vi "Save Image.vi"(8 "error in (no error)":errorcluster, 11 "Save Image in":refnum<class "Save Image.lvclass">) -> (0 "error out":errorcluster, 3 "Save Image out":refnum<class "Save Image.lvclass">)   [LabVIEW 2018, in "Save Image.lvclass"]
doc: "Save image using the Python Toolkit"
uses:
  Save Image.lvclass
  Save Image.lvclass/Save Image.ctl
  Log File/Log File.lvclass/Log File.ctl
  Channel/Channel.lvclass
  Log File/Log File.lvclass
  Python Toolkit/Python Toolkit.lvclass
  Sim_CCD/Sim_CCD.lvclass
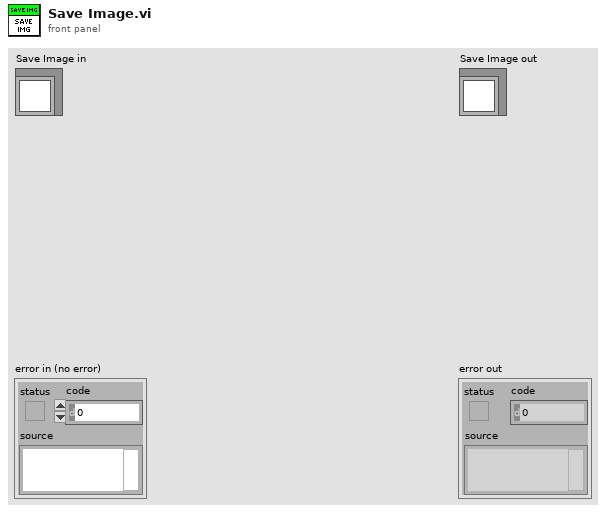
[diagram p1: front panel]
types:
  T1 = cluster{"CCD":string, "GUI":string, "ICS":string, "TCS":string, "FOCUSER":string, "WSTATION":string, "GENERAL KW":string}
  T2 = cluster{"Image path":path, "Channel":u8, "ACS mode":u16, "Log file path":path, "log level":u16}
  T3 = cluster{"CYCLES_DONE":u16, "LAST_IMAGE_NAME":string, "USED_DISK_SPACE":u16, "IMAGE_INDEX":u32, "acquisition error":bool}
  T4 = cluster{"State Machine.lvclass":refnum<class "State Machine.lvclass">, "RxTx.lvclass":refnum<class "RxTx.lvclass">, "Save_Header_RxTx.lvclass":refnum<class "RxTx.lvclass">, "Status SM.lvclass":refnum<class "State Machine.lvclass">, "Status RxTx.lvclass":refnum<class "RxTx.lvclass">, "servers array":refnum<class "Server.lvclass">[], "Events log file.lvclass":refnum<class "Log File.lvclass">, "Errors log file.lvclass":refnum<class "Log File.lvclass">, "Keywords log file.lvclass":refnum<class "Log File.lvclass">, "Sim_CCD.lvclass":refnum<class "Sim_CCD.lvclass">}
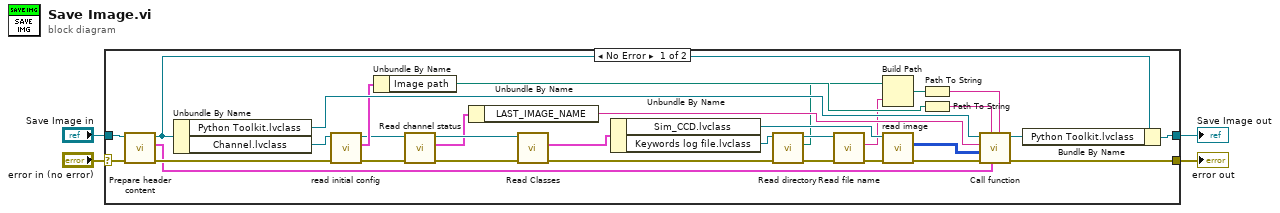
[diagram p0: block diagram]
diagram:
  n1 = case shown="No Error" "error in (no error)" {
    selector: "error in (no error)" -> [w30 w37]
    tunnel: [w11 w37] -> w1
    tunnel: [w36 w38] -> w2
    tunnel: "Save Image in" -> [w32 w38]
    frame No Error {
      n2 = call "Prepare header content.vi"("error in (no error)"=w30, "Save Image in"=w32) -> ("error out"=w28:errorcluster, "cluster of jsons 2"=w22:T1, "Save Image out"=w31:refnum<class "Save Image.lvclass">)  [unwired: 7 in]
      n3 = Unbundle By Name(w31) -> ("Python Toolkit.lvclass"=w35:refnum<class "Python Toolkit.lvclass">, "Channel.lvclass"=w29:refnum<class "Channel.lvclass">)
      n4 = call-dynamic "read initial config.vi"("error in (no error)"=w28, "Channel in"=w29) -> ("error out"=w6:errorcluster, "Configuration to initialize ACS"=w27:T2, "Channel out"=w9:refnum<class "Channel.lvclass">)  [unwired: 7 in]
      n5 = Unbundle By Name(w27) -> ("Image path"=w26:path)
      n6 = call-dynamic "Read channel status.vi"("error in (no error)"=w6, "Channel in"=w9) -> ("error out"=w7:errorcluster, "channel status"=w5:T3, "Channel out"=w8:refnum<class "Channel.lvclass">)  [unwired: 7 in]
      n7 = Unbundle By Name(w5) -> ("LAST_IMAGE_NAME"=w24:string)
      n8 = call-dynamic "Read Classes.vi"("error in (no error)"=w7, "Channel in"=w8) -> ("error out"=w21:errorcluster, "Classes"=w20:T4)  [unwired: 7 in, 1 out]
      n9 = Unbundle By Name(w20) -> ("Sim_CCD.lvclass"=w19:refnum<class "Sim_CCD.lvclass">, "Keywords log file.lvclass"=w10:refnum<class "Log File.lvclass">)
      n10 = call "Read directory.vi"("error in (no error)"=w21, "Log File in"=w10) -> ("error out"=w18:errorcluster, "directory"=w16:path, "Log File out"=w17:refnum<class "Log File.lvclass">)  [unwired: 7 in]
      n11 = call-dynamic "Read file name.vi"("error in (no error)"=w18, "Log File in"=w17) -> ("error out"=w33:errorcluster, "file name"=w15:string)  [unwired: 7 in, 1 out]
      n12 = Build Path(base path=w16, name or relative path=w15) -> (appended path=w14:path)
      n13 = call "read image.vi"("error in (no error)"=w33, "CCDCamera in"=w19) -> ("error out"=w34:errorcluster, "Image Graph"=w23:u16[][])  [unwired: 7 in, 1 out]
      n14 = Path To String(path=w14) -> (string=w13:string)
      n15 = Path To String(path=w26) -> (string=w25:string)
      n16 = call "Call function.vi"("log file path"=w13, "cluster of jsons"=w22, "night dir"=w25, "error in (no error)"=w34, "Array"=w23, "file name"=w24, "Python Toolkit in"=w35) -> ("error out"=w11:errorcluster, "Python Toolkit out"=w12:refnum<class "Python Toolkit.lvclass">)  [unwired: 3 in]
      n17 = Bundle By Name(cluster=w31, "Python Toolkit.lvclass"=w12) -> (w36:refnum<class "Save Image.lvclass">)
    }
    frame Error {
    }
  }
  "error out" <- w1
  "Save Image out" <- w2
